vi "GetFirstScreen.vi"(8 "error in (no error)":errorcluster, 11 "AboutScreen in":refnum<class "AboutScreen.lvclass">) -> (0 "error out":errorcluster, 2 "Array":u32[][](array[numeric]), 3 "AboutScreen out":refnum<class "AboutScreen.lvclass">)   [LabVIEW 2019, in "RT_Game.lvlib" / "AboutScreen.lvclass"]
uses:
  AboutScreen.lvclass
  Engine/Engine.lvclass
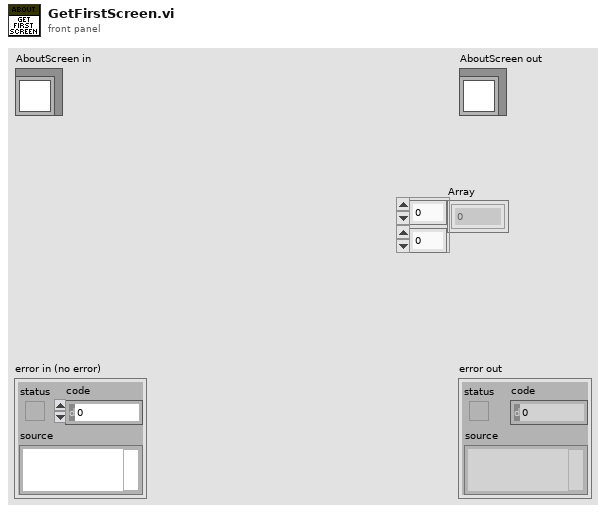
[diagram p1: front panel]
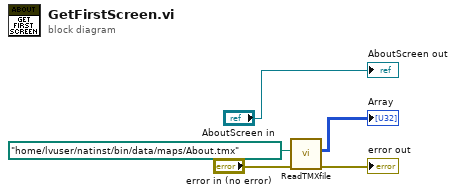
[diagram p0: block diagram]
diagram:
  n1 = call "ReadTMXfile.vi"("error in (no error)"="error in (no error)", "path to tmx-file (created with Tiles2D)"=path "/home/lvuser/natinst/bin/data/maps/About.tmx") -> ("error out"=→"error out":errorcluster, "Tilenumbers"=→"Array":u32[][])  [unwired: 8 in]
  "AboutScreen out" <- "AboutScreen in"
